vi "总磷氨氮MB_api.vi"(6 "Slave ID":u8=1, 7 "STEP":enum16{"open", "read", "write", "close"}(ring)=enum."read", 8 "Error in":errorcluster caption="Error in (no error)", 9 "values":u16[](array[numeric]), 10 "quantity":u16, 11 "starting address":u16 format="%04xH") -> (0 "error out":errorcluster, 1 "MB session out":refnum<class "MB_Master.lvclass">, 2 "输出簇":T1, 3 "Registers":u16[](array[numeric]))   [LabVIEW 2016, in "斯坦道仪器.lvlib"]
uses:
  <vilib>/Plasmionique/MB Master/MB_Master/MB_Master.lvclass
  <vilib>/Plasmionique/MB Master/MB_ADU/MB_ADU.lvclass/MB_ADU.ctl
  <vilib>/Plasmionique/MB Master/MB_ADU/Read RX Data.vi
  <vilib>/Plasmionique/MB Master/MB_ADU/Read RX Timestamp.vi
  <vilib>/Plasmionique/MB Master/MB_ADU/Read Slave ID.vi
  <vilib>/Plasmionique/MB Master/MB_ADU/Read TX Data.vi
  <vilib>/Plasmionique/MB Master/MB_ADU/Read TX Timestamp.vi
  <vilib>/Plasmionique/MB Master/MB_Master_Serial/MB_Master_Serial.lvclass
  C:/Program Files (x86)/National Instruments/LabVIEW 2016/vi.lib/Plasmionique/MB Master/MB_Master/MB_Master.lvclass
  <vilib>/Plasmionique/MB Master/MB_ADU/MB_ADU.lvclass
  <vilib>/Plasmionique/MB Master/MB Master.lvlib
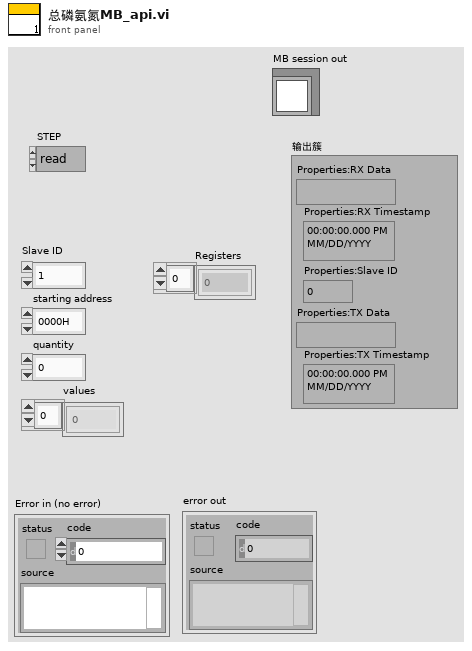
[diagram p1: front panel]
types:
  T1 = cluster{"Properties:RX Data":string, "Properties:RX Timestamp":timestamp, "Properties:Slave ID":u8, "Properties:TX Data":string, "Properties:TX Timestamp":timestamp}
  T2 = cluster{"baud rate (bps)":u32, "stop bits":u16, "parity":u16, "flow control":u16, "timeout":u32, "retries":i32}
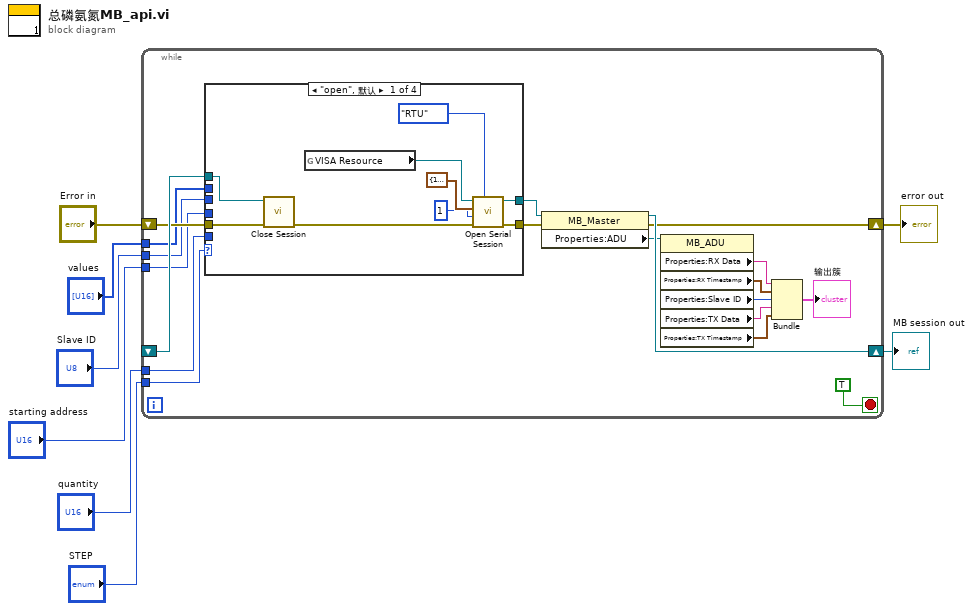
[diagram p0: block diagram]
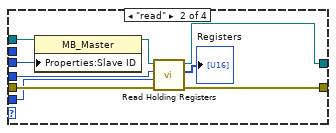
[diagram p2: hidden frame]
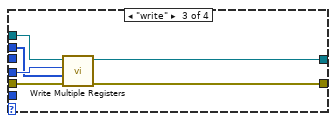
[diagram p3: hidden frame]
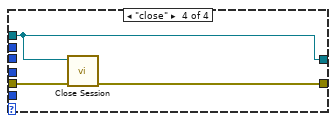
[diagram p4: hidden frame]
diagram:
  n1 = while {
    shift-right: [w20] -> w1
    shift-left: _ -> [w27]
    shift-right: [w18] -> w7
    shift-left: "Error in" -> [w26]
    tunnel: "Slave ID" -> [w25]
    tunnel: "starting address" -> [w24]
    tunnel: "quantity" -> [w23]
    tunnel: "STEP" -> [w22]
    tunnel: "values" -> [w10]
    stop <- TRUE stop-if-true
    n2 = case shown="\"open\", 默认" w22 {
      tunnel: w27 -> [w31 w38 w49 w52]
      tunnel: w26 -> [w30 w45 w51 w54]
      tunnel: [w32 w44 w48 w52] -> w21
      tunnel: [w34 w43 w50 w53] -> w19
      tunnel: w25 -> [_ w41 _ _]
      tunnel: w24 -> [_ w40 w47 _]
      tunnel: w23 -> [_ w39 _ _]
      tunnel: w10 -> [_ _ w46 _]
      frame "open", Default {
        n3 = call-dynamic "Close Session.vi"("error in (no error)"=w30, "MB session in"=w31) -> ("error out"=w29:errorcluster)  [unwired: 9 in]
        n4 = global read "VAR总磷氨氮全局变量.vi" "VISA Resource"() -> (w28:refnum<visa-resource-name>)
        n5 = call <vilib>:"Open Serial Session.vi"("Mode (RTU)"=enum16{"RTU", "ASCII"}."RTU", "Error in"=w29, "Slave ID"=u8 1, "Serial Config"=T2 {"baud rate (bps)"=115200, "stop bits"=10, "parity"=0, "flow control"=0, "timeout"=100, "retries"=1}, "VISA Resource"=w28) -> ("Error out"=w34:errorcluster, "MB_Serial session"=w32:refnum<class "MB_Master_Serial.lvclass">)  [unwired: 5 in]
      }
      frame "read" {
        n6 = property class="MB_Master"(reference=w38, "Properties:Slave ID"=w41) -> (reference out=w37:refnum<class "MB_Master.lvclass">)  [unwired: 1 in, 1 out]
        n7 = call <vilib>:"Read Holding Registers.vi"("error in (no error)"=w45, "quantity"=w39, "starting address"=w40, "MB session in"=w37) -> ("error out"=w43:errorcluster, "Registers"=→"Registers":u16[], "MB session out"=w44:refnum<class "MB_Master.lvclass">)  [unwired: 5 in]
      }
      frame "write" {
        n8 = call <vilib>:"Write Multiple Registers.vi"("error in (no error)"=w51, "values"=w46, "starting address"=w47, "MB session in"=w49) -> ("error out"=w50:errorcluster, "MB session out"=w48:refnum<class "MB_Master.lvclass">)  [unwired: 6 in]
      }
      frame "close" {
        n9 = call-dynamic "Close Session.vi"("error in (no error)"=w54, "MB session in"=w52) -> ("error out"=w53:errorcluster)  [unwired: 9 in]
      }
    }
    n10 = property class="MB_Master"(reference=w21, error in=w19) -> (reference out=w20:refnum<class "MB_Master.lvclass">, error out=w18:errorcluster, "Properties:ADU"=w17:refnum<class "MB_ADU.lvclass">)
    n11 = property class="MB_ADU"(reference=w17) -> ("Properties:RX Data"=w16:string, "Properties:RX Timestamp"=w15:timestamp, "Properties:Slave ID"=w14:u8, "Properties:TX Data"=w13:string, "Properties:TX Timestamp"=w12:timestamp)  [unwired: 1 in, 2 out]
    n12 = Bundle("Properties:RX Data"=w16, "Properties:RX Timestamp"=w15, "Properties:Slave ID"=w14, "Properties:TX Data"=w13, "Properties:TX Timestamp"=w12) -> (→"输出簇":T1)  [unwired: 1 in]
  }
  "error out" <- w7
  "MB session out" <- w1
